vi "Initialize (SubVI).vi"(0 "Communications Port":refnum<visa-resource-name>="COM3", 2 "InterfaceType":i32(ring)=1 items=["Usb", "Serial", "Ethernet", "Unconnected"], 5 "error in (no error)":errorcluster) -> (12 "IsConnected":bool, 14 "ILabVIEW":refnum<k24>, 19 "error out":errorcluster)   [LabVIEW 2017]
doc: "Establishes communication with the <B>Watlow Standard Bus</B> product. Call this VI before calling other instrument driver VIs for this product. Generally, you need to call the <B>Initialize VI</B> only once at the beginning of an application.\n\nThis VI Driver set supports the following communication protocols. The user will select the type from the <B> InterfaceType</B> Control.\n\n<B>Serial</B> - RS 485 Communications - The user will select the serial comms port available in the Communicaitons Port Control (COM3, COM4)\n<B> USB </B> - The user will enter the Unit Serial Number in the Communications Control (Example: 12345). Currently no Watlow products support this protocol. Contact Watlow for avabilabity.\n<B> Ethernet</B> - The user will enter the controls IP address in the Communications Port Control. (Example: 192.168.0.222).\n\n<B> IsConnected</B> control tells the user that a successful communication connection has been established and may continue with any read/write operations. Use this control as an indication that the VI properly initialized.\n<B> Interface Found </B> control tells the user that the selected Interface was found. This does not indicate that it connected to the device. Use the <B> IsConnected </B> control as an indication that the VI properly initialized."
uses:
  dll/Watbus.dll
  <vilib>/regexp/Match Regular Expression.xnode
panel:
  out "Description":string
  out "size(s)":i32
  out "Interface":i32
  # "Std Bus Initialize"
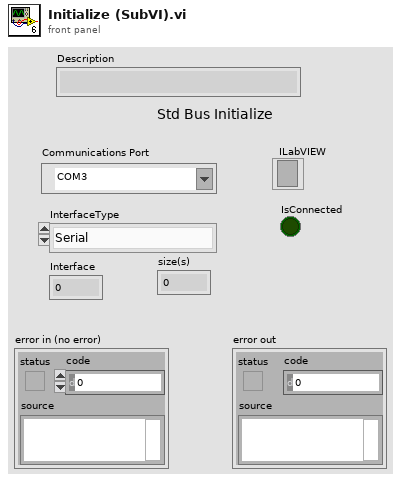
[diagram p1: front panel]
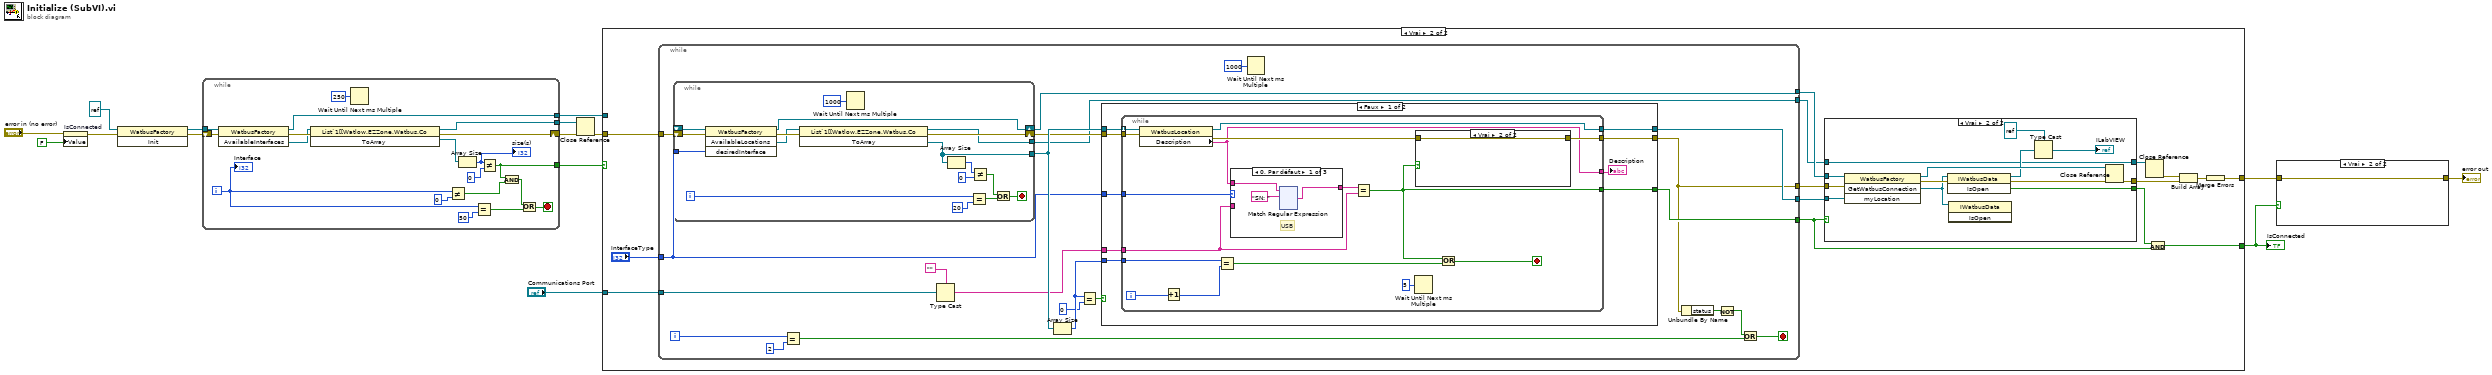
[diagram p0: block diagram]
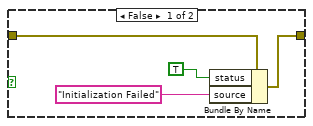
[diagram p2: hidden frame]
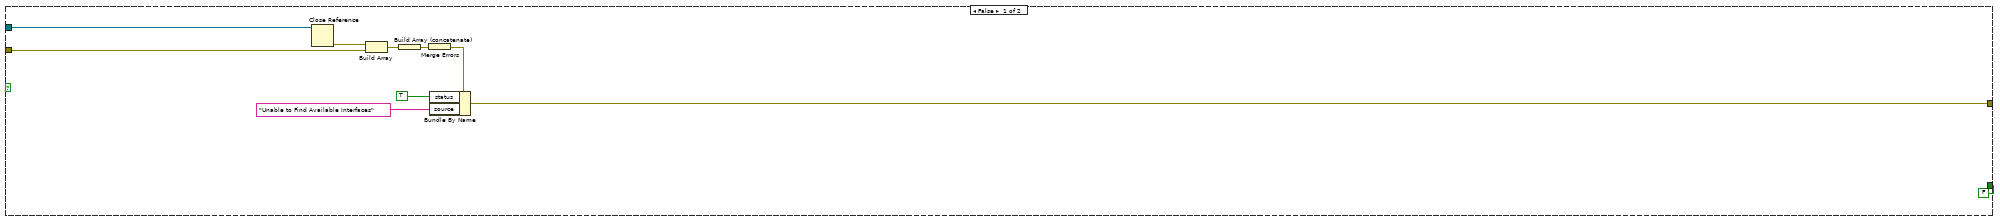
[diagram p3: hidden frame]
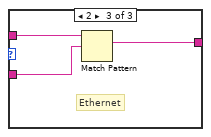
[diagram p5: hidden frame]
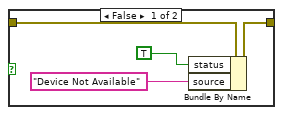
[diagram p6: hidden frame]
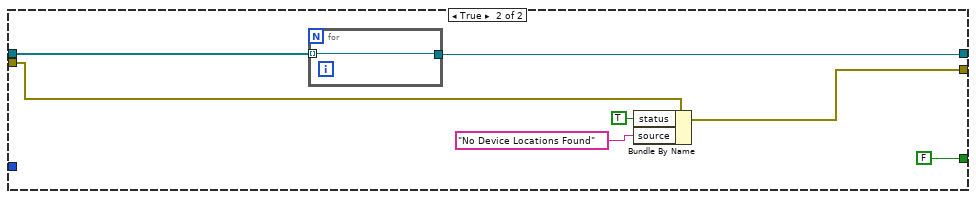
[diagram p7: hidden frame]
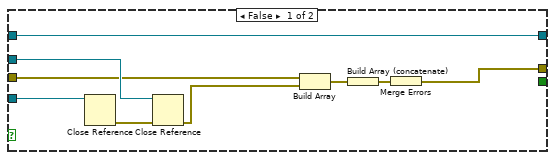
[diagram p8: hidden frame]
diagram:
  n1 = property on="IsConnected" class="Bool (strict)"(error in="error in (no error)", "Value"=FALSE ("IsConnected")) -> (error out=w14:errorcluster)  [unwired: 1 in, 1 out]
  n2 = invoke class="WatbusFactory" method="Init"(reference=refnum<k24> refnum ("ConstructClient"), error in=w14) -> (reference out=w10:refnum<k24>, error out=w9:errorcluster)  [unwired: 1 in, 1 out]
  n3 = while {
    shift-right: [w28] -> w12
    shift-left: w9 -> [w32]
    tunnel: [w18] -> w8
    tunnel: w10 -> [w33]
    tunnel: [w34] -> w6
    tunnel: [w16] -> w11
    i -> [w24]
    stop <- w21 stop-if-true
    n4 = invoke class="WatbusFactory" method="AvailableInterfaces"(reference=w33, error in=w32) -> (reference out=w34:refnum<k24>, error out=w30:errorcluster, "AvailableInterfaces"=w29:refnum<k24>)  [unwired: 1 in]
    n5 = invoke class="List`1[[Watlow.EZZone.Watbus.Co" method="ToArray"(reference=w29, error in=w30) -> (reference out=w16:refnum<k24>, error out=w28:errorcluster, "ToArray"=w17:refnum<k24>[])  [unwired: 1 in]
    n6 = Wait Until Next ms Multiple(millisecond multiple=u32 250) -> ()  [unwired: 1 out]
    n7 = Not Equal?(x=w24, y=0) -> (x != y?=w25:bool)
    n8 = Array Size(array=w17) -> (size(s)=w19:i32)
    "size(s)" <- w19
    n9 = Equal?(x=w24, y=50) -> (x = y?=w23:bool)
    n10 = Not Equal?(x=w19, y=0) -> (x != y?=w18:bool)
    n11 = And(x=w18, y=w25) -> (x .and. y?=w27:bool)
    n12 = Or(x=w27, y=w23) -> (x .or. y?=w21:bool)
    "Interface" <- w24
  }
  n13 = Close Reference(reference=w11, error in (no error)=w12) -> (error out=w7:errorcluster)
  n14 = case shown="Vrai" w8 {
    tunnel: [w37 w52] -> w2
    tunnel: w7 -> [w38 w51]
    tunnel: w6 -> [w39 _]
    tunnel: [FALSE ("IsOpen") w45] -> w3
    tunnel: "Communications Port" -> [_ w50]
    frame False {
      n15 = Close Reference(reference=w39) -> (error out=w40:errorcluster)  [unwired: 1 in]
      n16 = Build Array(w40, w38) -> (w44:errorcluster[])
      n17 = Build Array (concatenate)(w44) -> (w35:errorcluster[])
      n18 = Merge Errors(w35) -> (w41:errorcluster)
      n19 = Bundle By Name(cluster=w41, "status"=TRUE, "source"="Unable to Find Available Interfaces") -> (w37:errorcluster)
    }
    frame True {
      n20 = while {
        tunnel: [w81] -> w59
        tunnel: [w68] -> w58
        tunnel: [w80] -> w57
        tunnel: [w74] -> w54
        tunnel: w51 -> [w73]
        tunnel: w50 -> [w71]
        tunnel: "InterfaceType" -> [w70]
        tunnel: [w69] -> w46
        i -> [w61]
        stop <- w64 stop-if-true
        n21 = while {
          tunnel: w70 -> [w242]
          tunnel: [w252] -> w79
          shift-right: [w253] -> w81
          shift-left: _ -> [w255]
          shift-right: [w254] -> w75
          shift-left: w73 -> [w249]
          tunnel: [w241] -> w74
          i -> [w245]
          stop <- w247 stop-if-true
          n22 = invoke class="WatbusFactory" method="AvailableLocations"(reference=w255, error in=w249, "desiredInterface"=w242) -> (reference out=w253:refnum<k24>, error out=w257:errorcluster, "AvailableLocations"=w256:refnum<k24>)  [unwired: 1 in, 1 out]
          n23 = invoke class="List`1[[Watlow.EZZone.Watbus.Co" method="ToArray"(reference=w256, error in=w257) -> (reference out=w241:refnum<k24>, error out=w254:errorcluster, "ToArray"=w252:refnum<k24>[])  [unwired: 1 in]
          n24 = Wait Until Next ms Multiple(millisecond multiple=u32 1000) -> ()  [unwired: 1 out]
          n25 = Array Size(array=w252) -> (size(s)=w250:i32)
          n26 = Equal?(x=w245, y=20) -> (x = y?=w244:bool)
          n27 = Not Equal?(x=w250, y=0) -> (x != y?=w248:bool)
          n28 = Or(x=w248, y=w244) -> (x .or. y?=w247:bool)
        }
        n29 = Equal?(x=w61, y=2) -> (x = y?=w63:bool)
        n30 = Type Cast(type="", x=w71) -> (*(type *) &x=w72:string)
        n31 = Array Size(array=w79) -> (size(s)=w78:i32)
        n32 = Equal?(x=w78, y=0) -> (x = y?=w76:bool)
        n33 = case shown="Faux" w76 {
          tunnel: [w84 w239] -> w68
          tunnel: [w90 w233] -> w80
          tunnel: w75 -> [w89 w238]
          tunnel: w70 -> [w88 _]
          tunnel: w78 -> [w87 _]
          tunnel: w79 -> [w86 w234]
          tunnel: [w85 FALSE] -> w69
          tunnel: w72 -> [w82 _]
          frame False {
            n34 = while {
              tunnel: w89 -> [w106]
              tunnel: w86 -> [w105] mode=indexing
              tunnel: w87 -> [w100]
              tunnel: w88 -> [w99]
              tunnel: [w91] -> w90
              tunnel: [w96] -> w85
              tunnel: [w94] -> w84
              tunnel: [w93] -> w83
              tunnel: w82 -> [w92]
              i -> [w101]
              stop <- w95 stop-if-true
              n35 = property class="WatbusLocation"(reference=w105, error in=w106) -> (reference out=w91:refnum<k24>, error out=w102:errorcluster, "Description"=w93:string)
              n36 = Increment(x=w101) -> (x+1=w103:i32)
              n37 = Equal?(x=w100, y=w103) -> (x = y?=w104:bool)
              n38 = case shown="0, Par défaut" w99 {
                tunnel: w93 -> [w108 w224 w227]
                tunnel: [w107 w224 w225] -> w98
                tunnel: w92 -> [_ _ w226]
                frame 0, Default {
                  # "USB"
                  n39 = xnode "Match Regular Expression"("chaîne en entrée"=w108, "expression régulière"="SN: " ("regular expression")) -> ("après la correspondance"=w107:string)  [unwired: 2 in, 6 out]
                }
                frame 1 {
                  # "Serial Comms"
                }
                frame 2 {
                  # "Ethernet"
                  n40 = Match Pattern(string=w227, regular expression=w226) -> (match substring=w225:string)  [unwired: 4 out]
                }
              }
              n41 = Equal?(x=w98, y=w92) -> (x = y?=w96:bool)
              n42 = Wait Until Next ms Multiple(millisecond multiple=u32 5) -> ()  [unwired: 1 out]
              n43 = case shown="Vrai" w96 {
                tunnel: w102 -> [w231 w232]
                tunnel: [w230 w232] -> w94
                frame False {
                  n44 = Bundle By Name(cluster=w231, "status"=TRUE, "source"="Device Not Available") -> (w230:errorcluster)
                }
                frame True {
                }
              }
              n45 = Or(x=w96, y=w104) -> (x .or. y?=w95:bool)
            }
            "Description" <- w83
          }
          frame True {
            n46 = for {
              tunnel: w234 -> [w240] mode=indexing
              tunnel: [w240] -> w233
            }
            n47 = Bundle By Name(cluster=w238, "status"=TRUE, "source"="No Device Locations Found") -> (w239:errorcluster)
          }
        }
        n48 = Wait Until Next ms Multiple(millisecond multiple=u32 1000) -> ()  [unwired: 1 out]
        n49 = Unbundle By Name(w68) -> ("status"=w66:bool)
        n50 = Not(x=w66) -> (.not. x?=w65:bool)
        n51 = Or(x=w65, y=w63) -> (x .or. y?=w64:bool)
      }
      n52 = case shown="Vrai" w46 {
        tunnel: [w263 w278] -> w55
        tunnel: w59 -> [w266 w277]
        tunnel: w58 -> [w265 w276]
        tunnel: w57 -> [w262 w275]
        tunnel: w54 -> [w259 w271]
        tunnel: [w259 w271] -> w53
        tunnel: [_ w269] -> w47
        frame False {
          n53 = Close Reference(reference=w262) -> (error out=w261:errorcluster)  [unwired: 1 in]
          n54 = Close Reference(reference=w266, error in (no error)=w261) -> (error out=w264:errorcluster)
          n55 = Build Array(w265, w264) -> (w260:errorcluster[])
          n56 = Build Array (concatenate)(w260) -> (w258:errorcluster[])
          n57 = Merge Errors(w258) -> (w263:errorcluster)
        }
        frame True {
          n58 = invoke class="WatbusFactory" method="GetWatbusConnection"(reference=w277, error in=w276, "myLocation"=w275) -> (reference out=w279:refnum<k24>, error out=w274:errorcluster, "GetWatbusConnection"=w267:refnum<k24>)  [unwired: 1 in, 1 out]
          n59 = invoke class="IWatbusData" method="IsOpen"(reference=w267, error in=w274) -> (reference out=w273:refnum<k24>, error out=w270:errorcluster, "IsOpen"=w269:bool)  [unwired: 1 in]
          n60 = invoke class="IWatbusData" method="IsOpen"(reference=w267) -> ()  [unwired: 2 in, 3 out]
          n61 = Type Cast(type=refnum<k24> refnum ("ConstructClient"), x=w273) -> (*(type *) &x=→"ILabVIEW":refnum<k24>)
          n62 = Close Reference(reference=w279, error in (no error)=w270) -> (error out=w278:errorcluster)
        }
      }
      n63 = Close Reference(reference=w53) -> (error out=w56:errorcluster)  [unwired: 1 in]
      n64 = And(x=w47, y=w46) -> (x .and. y?=w45:bool)
      n65 = Build Array(w56, w55) -> (w48:errorcluster[])
      n66 = Merge Errors(w48) -> (w52:errorcluster)
    }
  }
  "IsConnected" <- w3
  n67 = case shown="Vrai" w3 {
    tunnel: w2 -> [w283 w284]
    tunnel: [w282 w284] -> w1
    frame False {
      n68 = Bundle By Name(cluster=w283, "status"=TRUE, "source"="Initialization Failed") -> (w282:errorcluster)
    }
    frame True {
    }
  }
  "error out" <- w1
